vi "Save_dialogue_number_ION.vi"() -> (0 "Температура 2":i32, 1 "Номер образца 2":i32, 2 "Номер сеанса 2":i32, 3 "Ион 2":string, 5 "OK Button 2":bool)   [LabVIEW 2013]
panel:
  in  "Ион":string
  in  "Номер сеанса":i32
  in  "Температура":i32
  in  "Номер образца":i32
  out "stop 2":bool
  in  "stop":bool
  in  "OK Button":bool
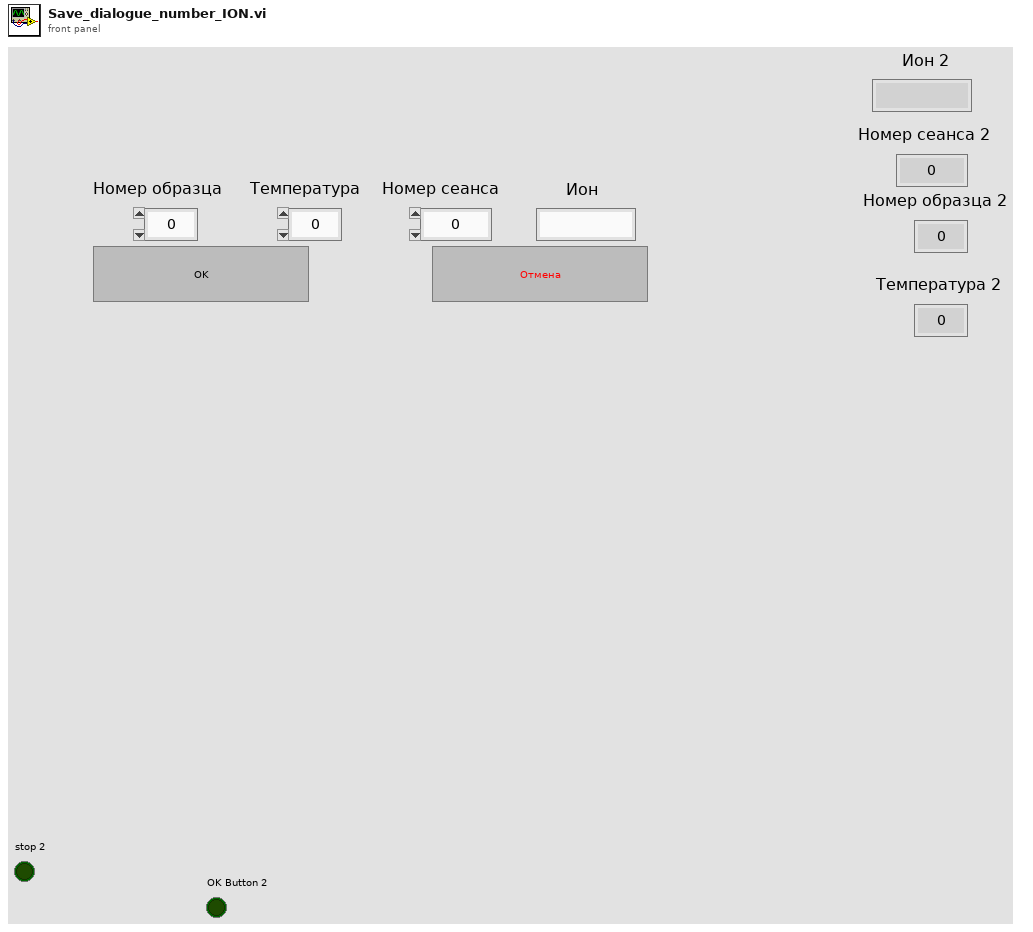
[diagram p1: front panel]
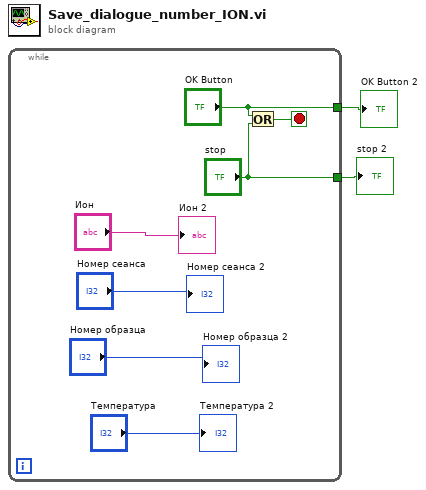
[diagram p0: block diagram]
diagram:
  n1 = while {
    tunnel: ["OK Button"] -> w2
    tunnel: ["stop"] -> w1
    stop <- w9 stop-if-true
    n2 = Or(x="OK Button", y="stop") -> (x .or. y?=w9:bool)
    "Номер образца 2" <- "Номер образца"
    "Температура 2" <- "Температура"
    "Номер сеанса 2" <- "Номер сеанса"
    "Ион 2" <- "Ион"
  }
  "OK Button 2" <- w2
  "stop 2" <- w1
